vi "PLC OPC Prototype.vi"() -> ()   [LabVIEW 2013]
uses:
  Sub VIs/OPC Engine/Controls/OPC Write Registers.ctl
  Sub VIs/OPC Engine/Controls/OPC Write Global Options.ctl
  Sub VIs/OPC Engine/Controls/OPC Read Registers.ctl
  Sub VIs/OPC Engine/Globals/OPC Engine Globals.vi
panel:
  out "Read Values":i32[](array[numeric])
  in  "OPC Write Register Array":T1[](array[typedef])=[enum."Air Leak Test Not Passed", enum."Repair Code Missing", enum."Estop Alarm Light"]
  in  "Write Values":i32[](array[numeric])=[1, 0, 1]
  in  "Read Registers":string[](array[string])=["[Master_PLC]DACS_TS1_Air_Leak_Test_Not_Passed", "[Master_PLC]DACS_TS1_Repair_Code_Missing", "[Master_PLC]DACS_TS1_Estop_Alarm_Light"]
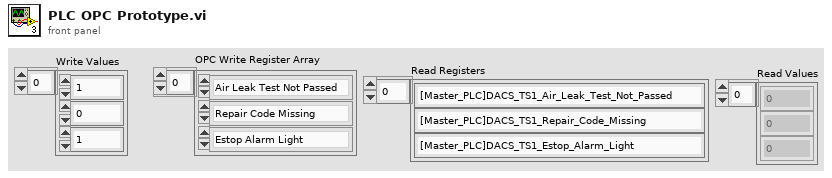
[diagram p1: front panel]
types:
  T1 = typedef "OPC Write Registers.ctl" = enum16{"DACS Alive", "DACS Ready to Run", "Load Fixture Request", "Fixture Ready Ack", "Serial Number Valid", "Unload Fixture Request", "Test Status", "Motor Present", "Serial Number Request for UUT", "Coupling Request", "Coupling Number Request", "At Coupling Change Position", "At Coupling Clear Position", "Coupling Load Complete Ack", "Serial Number Status", "Locator Position", "Fixture Block", "Nametag Location", "Air Leak Test Not Passed", "Repair Code Missing", "Estop Alarm Light"}
  T2 = enum16{"Read", "Write", "ReadWrite", "BufferedRead", "BufferedReadWrite"}
  T3 = typedef "OPC Write Global Options.ctl" = enum16{"Init", "Write Value", "Write Array", "Read Value", "Read Array", "Read All"}
  T4 = typedef "OPC Read Registers.ctl" = enum16{"Load Request Ack", "UUT Serial Number", "Fixture Ready Request", "Unload Request Ack", "Load Complete", "UnLoad Complete", "Read Motor Speed", "Read Milking Motor Speed", "Coupling Ack", "Coupling Load Complete", "Coupling Change Position Request", "Coupling Clear Position Request", "Load Coupling Request", "Coupling Load Fail", "UUT Serial Number Verify Request", "Serial number at scanner", "Other UUT Serial number", "Master PLC Alive"}
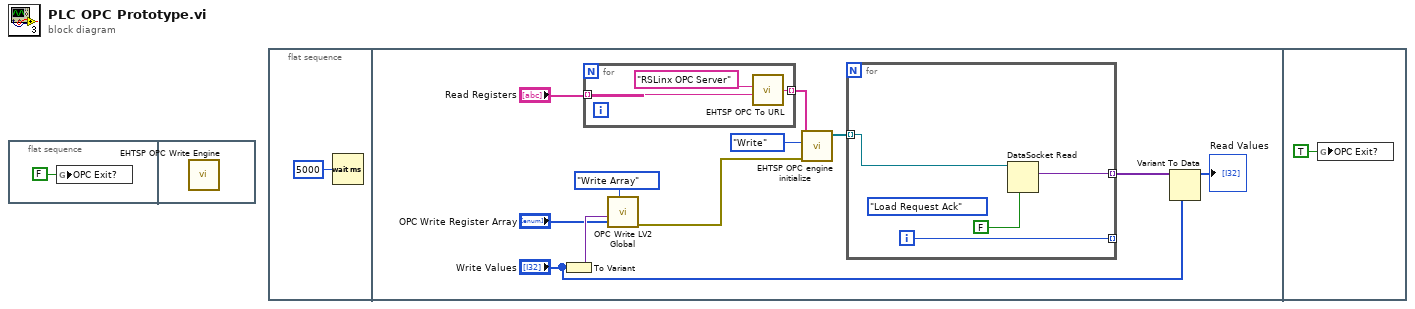
[diagram p0: block diagram]
diagram:
  n1 = flat-sequence {
    frame #0 {
      n2 = global write "OPC Engine Globals.vi" "OPC Exit?"(FALSE ("OPC Exit?")) -> ()
    }
    frame #1 {
      n3 = call "EHTSP OPC Write Engine.vi"() -> ()  [unwired: 11 in, 1 out]
    }
  }
  n4 = flat-sequence {
    frame #0 {
      n5 = Wait (ms)(milliseconds to wait=u32 5000) -> ()  [unwired: 1 out]
    }
    frame #1 {
      n6 = To Variant(anything="Write Values") -> (Variant=w12:variant)
      n7 = for {
        tunnel: "Read Registers" -> [w20] mode=indexing
        tunnel: [w19] -> w11 mode=indexing
        n8 = call "EHTSP OPC To URL.vi"("Item Name"=w20, "Server Name"="RSLinx OPC Server") -> ("URL"=w19:string)  [unwired: 4 in]
      }
      n9 = call "OPC Write LV2 Global.vi"("Options"=OPC_Write_Global_Options."Write Array", "OPC value"=w12, "OPC Write Register Array"="OPC Write Register Array") -> ("error out"=w3:errorcluster)  [unwired: 4 in, 4 out]
      n10 = call "EHTSP OPC engine initialize.vi"("error in (no error)"=w3, "mode"=T2."Write", "URLs"=w11) -> ("Connection ids"=w8:refnum<k13>[])  [unwired: 7 in, 1 out]
      n11 = for {
        tunnel: [w17] -> w7 mode=indexing
        tunnel: [w15] -> _ mode=indexing
        tunnel: w8 -> [w14] mode=indexing
        i -> [w15]
        (unwired) OPC_Read_Registers."Load Request Ack" ("Read Register")
        n12 = DataSocket Read(6:FALSE ("wait for updated value (T)"), 11:w14) -> (2:w17:variant)  [unwired: 3 in, 6 out]
      }
      n13 = Variant To Data(type="Write Values", Variant=w7) -> (data=→"Read Values":i32[])  [unwired: 1 in, 1 out]
    }
    frame #2 {
      n14 = global write "OPC Engine Globals.vi" "OPC Exit?"(TRUE ("OPC Exit?")) -> ()
    }
  }
